vi "LDF Get Frame Signal Name.vi"(7 "pSignalName":string, 9 "index":i32, 10 "pFrameName":string, 11 "LDFHandle":u64) -> (2 "pFrameName out":string, 3 "function return":i32, 5 "pSignalName out":string)   [LabVIEW 2010, in "ldf_parser.lvlib"]
doc: "int WINAPI LDF_GetFrameSignalName(long long LDFHandle, char* pFrameName, int index, char* pSignalName);"
uses:
  ldf_parser.lvlib
  USB2XXX/trunk/USB2XXX/USB2XXX/vs2019/Release/USB2XXX.dll
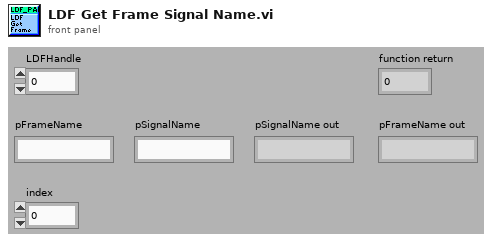
[diagram p1: front panel]
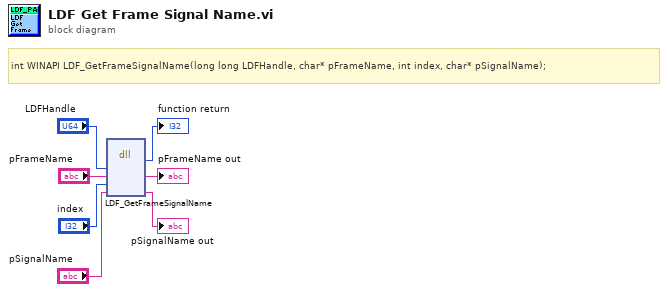
[diagram p0: block diagram]
diagram:
  # "int WINAPI LDF_GetFrameSignalName(long long LDFHandle, char* pFrameName, int index, char* pSignalName);"
  n1 = dll-call lib="E:/Projects/USB2XXX/trunk/USB2XXX/USB2XXX/vs2019/Release/USB2XXX.*" fn="LDF_GetFrameSignalName"("LDFHandle"="LDFHandle", "pFrameName"="pFrameName", "index"="index", "pSignalName"="pSignalName") -> (→"function return":i32, "pFrameName"=→"pFrameName out":string, "pSignalName"=→"pSignalName out":string)  [unwired: 5 in, 2 out]
